vi "Seconds to Hours-Minutes.vi"(11 "Time in Seconds":dbl) -> (1 "Numeric Control 3":dbl, 2 "Numeric Control 2":dbl, 3 "Numeric Control":dbl)   [LabVIEW 2015]
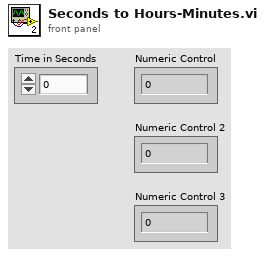
[diagram p1: front panel]
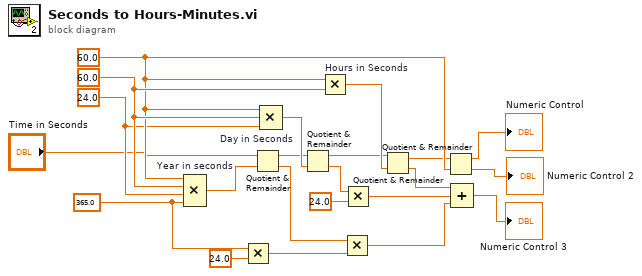
[diagram p0: block diagram]
diagram:
  w20 = 365.0
  w8 = 24.0
  w18 = 60.0
  w17 = 60.0
  n1 = Compound Arithmetic op=MULTIPLY "Year in seconds"(w17, w18, w8, w20) -> (w2:dbl)
  n2 = Multiply(x=w20, y=24.0) -> (x*y=w22:dbl)
  n3 = Quotient & Remainder(x="Time in Seconds", y=w2) -> (x-y*floor(x/y)=w3:dbl, floor(x/y)=w6:dbl)
  n4 = Compound Arithmetic op=MULTIPLY "Day in Seconds"(w17, w18, w8) -> (w7:dbl)
  n5 = Quotient & Remainder(x=w3, y=w7) -> (x-y*floor(x/y)=w4:dbl, floor(x/y)=w9:dbl)
  n6 = Multiply "Hours in Seconds"(x=w17, y=w18) -> (x*y=w5:dbl)
  n7 = Multiply(x=w6, y=w22) -> (x*y=w13:dbl)
  n8 = Multiply(x=w9, y=24.0) -> (x*y=w12:dbl)
  n9 = Quotient & Remainder(x=w4, y=w5) -> (x-y*floor(x/y)=w10:dbl, floor(x/y)=w11:dbl)
  n10 = Quotient & Remainder(x=w10, y=w17) -> (x-y*floor(x/y)=→"Numeric Control":dbl, floor(x/y)=→"Numeric Control 2":dbl)
  n11 = Compound Arithmetic op=ADD(w11, w12, w13) -> (→"Numeric Control 3":dbl)
